vi "StopProcess.vi"(0 "reference in":refnum<class "TestView_Base.lvclass">, 2 "ms timeout (-1)":i32=-1, 5 "error in (no error)":errorcluster) -> (14 "reference out":refnum<class "TestView_Base.lvclass">, 19 "error out":errorcluster)   [LabVIEW 2017]
uses:
  TestView_Base.lvclass
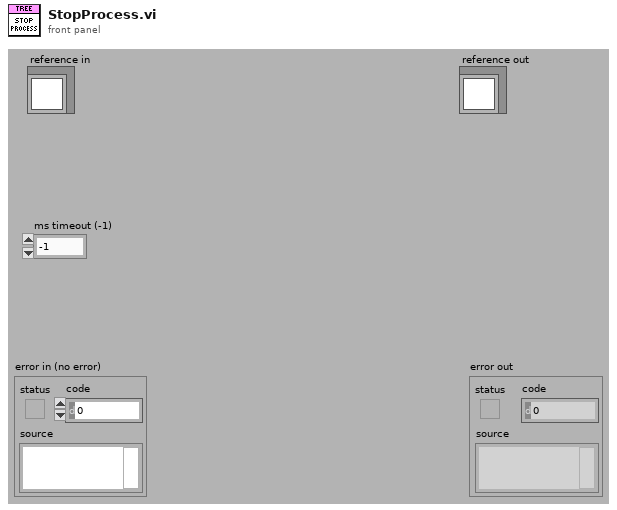
[diagram p1: front panel]
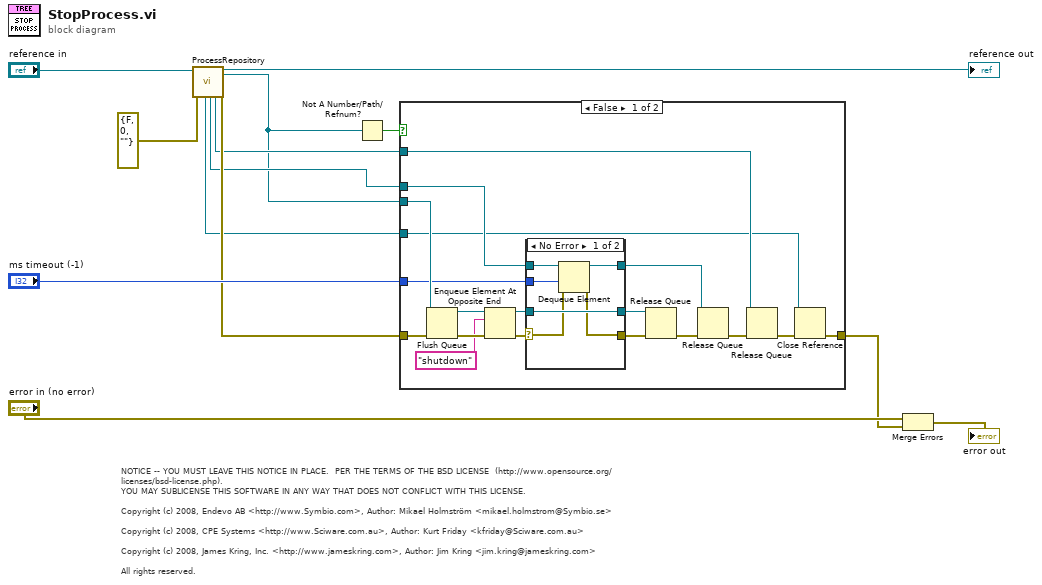
[diagram p0: block diagram]
diagram:
  # "NOTICE -- YOU MUST LEAVE THIS NOTICE IN PLACE.  PER THE TERMS OF THE BSD LICENSE  (http://www.opensource.org/licenses/bsd-license.php).\nYOU MAY SUBLICENSE THIS SOFTWARE IN ANY WAY THAT DOES NOT CONFLICT WITH THIS LICENSE.\n\nCopyright (c) 2008, Endevo AB <http://www.Symbio.com>, Author: Mikael Holmström <mikael.holmstrom@Symbio.se>\n\nCopyright (c) 2008, CPE Systems <http://www.Sciware.com.au>, Author: Kurt Friday <kfriday@Sciware.com.au>\n\nCopyright (c) 2008, James Kring, Inc. <http://www.jameskring.com>, Author: Jim Kring <jim.kring@jameskring.com>\n\nAll rights reserved."
  n1 = call "ProcessRepository.vi"("reference in"="reference in", "error in (no error)"=errorcluster {"status"=FALSE, "code"=0, "source"=""}) -> ("ProcessViRef"=w4:refnum<vi>, "ProcessSyncQueue"=w6:refnum<queue>, "FromProcessQueue"=w5:refnum<queue>, "reference out"=→"reference out":refnum<class "TestView_Base.lvclass">, "ToProcessQueue"=w2:refnum<queue>, "error out"=w7:errorcluster)  [unwired: 11 in, 1 out]
  n2 = Not A Number/Path/Refnum?(number/path/refnum=w2) -> (NaN/Path/Refnum?=w1:bool)
  n3 = case shown="False" w1 {
    tunnel: w6 -> [w26 _]
    tunnel: w7 -> [w28 w41]
    tunnel: [w21 w41] -> w11
    tunnel: w2 -> [w31 _]
    tunnel: "ms timeout (-1)" -> [w20 _]
    tunnel: w5 -> [w18 _]
    tunnel: w4 -> [w17 _]
    frame False {
      n4 = Flush Queue(queue=w31, error in (no error)=w28) -> (queue out=w29:refnum<queue>, error out=w30:errorcluster)  [unwired: 1 out]
      n5 = Enqueue Element At Opposite End(queue=w29, element="shutdown", error in (no error)=w30) -> (queue out=w25:refnum<queue>, error out=w19:errorcluster)  [unwired: 1 in, 1 out]
      n6 = case shown="No Error" w19 {
        tunnel: [w33 w40] -> w24
        tunnel: w26 -> [w36 w38]
        tunnel: [w37 w39] -> w23
        tunnel: w25 -> [w37 w39]
        tunnel: w20 -> [w35 _]
        selector: w19 -> [w34 w40]
        tunnel: [w32 w38] -> w15
        frame No Error {
          n7 = Dequeue Element(queue=w36, timeout in ms (-1)=w35, error in (no error)=w34) -> (queue out=w32:refnum<queue>, error out=w33:errorcluster)  [unwired: 2 out]
        }
        frame Error {
        }
      }
      n8 = Release Queue(queue=w23, error in (no error)=w24) -> (error out=w16:errorcluster)  [unwired: 1 in, 2 out]
      n9 = Release Queue(queue=w15, error in (no error)=w16) -> (error out=w14:errorcluster)  [unwired: 1 in, 2 out]
      n10 = Release Queue(queue=w18, error in (no error)=w14) -> (error out=w22:errorcluster)  [unwired: 1 in, 2 out]
      n11 = Close Reference(reference=w17, error in (no error)=w22) -> (error out=w21:errorcluster)
    }
    frame True {
    }
  }
  n12 = Merge Errors("error in (no error)", w11) -> (→"error out":errorcluster)
